vi "Update Output.vi"(8 "error in (no error)":errorcluster, 11 "Bioreactor in":refnum<class "Bioreactor.lvclass">) -> (0 "error out":errorcluster, 3 "Bioreactor out":refnum<class "Bioreactor.lvclass">)   [LabVIEW 2012]
uses:
  Bioreactor.lvclass
  Bioreactor.lvclass/Bioreactor.ctl
  Read Loop Name.vi
  Read Control Value.vi
  Read DVR.vi
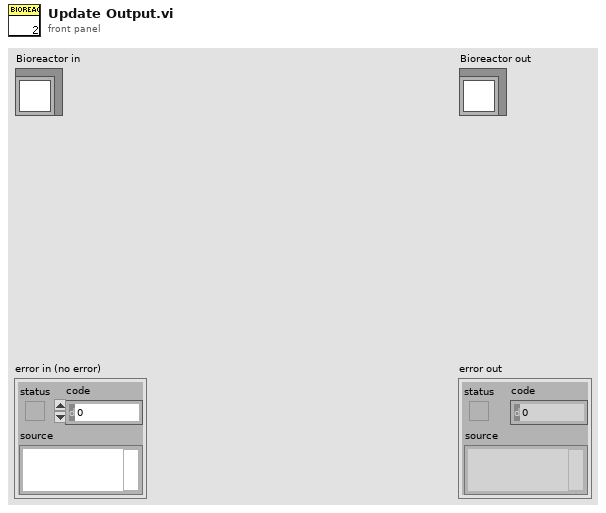
[diagram p1: front panel]
types:
  T1 = cluster{"Name":string, "Value":dbl, "Setpoint":dbl, "Output":dbl}[]
  T2 = cluster{"Name":string, "Value":dbl, "Setpoint":dbl, "Output":dbl}
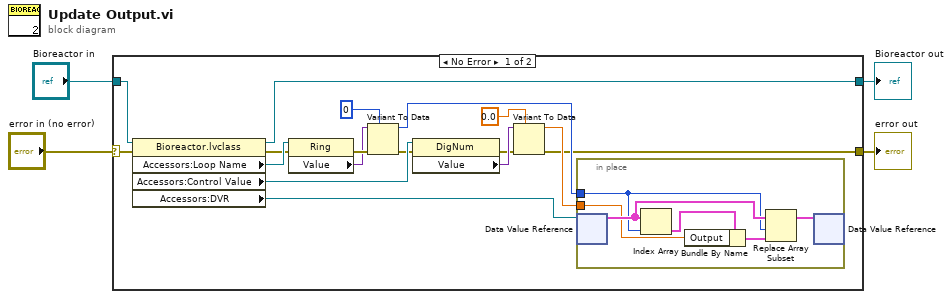
[diagram p0: block diagram]
diagram:
  n1 = case shown="No Error" "error in (no error)" {
    selector: "error in (no error)" -> [w11 w29]
    tunnel: [w6 w29] -> w2
    tunnel: [w9 w28] -> w1
    tunnel: "Bioreactor in" -> [w10 w28]
    frame No Error {
      n2 = property class="Bioreactor.lvclass"(reference=w10, error in=w11) -> (reference out=w9:refnum<class "Bioreactor.lvclass">, error out=w8:errorcluster, "Accessors:Loop Name"=w18:refnum<vi>, "Accessors:Control Value"=w14:refnum<vi>, "Accessors:DVR"=w5:refnum<data-value>)
      n3 = property class="Ring"(reference=w18, error in=w8) -> (error out=w21:errorcluster, "Value"=w20:variant)  [unwired: 1 out]
      n4 = Variant To Data(error in=w21, type=0, Variant=w20) -> (data=w13:i32, error out=w7:errorcluster)
      n5 = property class="DigNum"(reference=w14, error in=w7) -> (error out=w15:errorcluster, "Value"=w16:variant)  [unwired: 1 out]
      n6 = Variant To Data(error in=w15, type=0.0, Variant=w16) -> (data=w12:dbl, error out=w6:errorcluster)
      n7 = in-place {
        in-place-border: w13 -> [w23]
        in-place-border: w12 -> [w25]
        n8 = in-place-dvr #1(w5) -> (w27:T1)  [unwired: 1 out]
        n9 = Index Array(array=w27, index=w23) -> (element=w26:T2)
        n10 = Bundle By Name(cluster=w26, "Output"=w25) -> (w24:T2)
        n11 = Replace Array Subset(array=w27, new element=w24, index=w23) -> (w22:T1)
        n12 = in-place-dvr #1(w22) -> ()  [unwired: 2 out]
      }
    }
    frame Error {
    }
  }
  "error out" <- w2
  "Bioreactor out" <- w1
